vi "grab, fill rect, set:get pixel.vi"() -> ()   [LabVIEW 2011]
uses:
  <userlib>/labvvis/Rectangle.ctl
  <userlib>/labvvis/RGBA Pixel.ctl
  <userlib>/labvvis/New Image/New Image (RGBA).vi
  <userlib>/labvvis/Set Pixel/Set Pixel (RGBA).vi
  <userlib>/labvvis/Get Pixel/Get Pixel (RGBA).vi
  <userlib>/labvvis/labvvis.lvlib
panel:
  in  "Set Pixel":u8
  out "Error":string
  in  "Set Pixel":T1
  out "Get Pixel":u8
  out "Get Pixel":T1
  in  "Rectangle":T2
  in  "stop":bool
  out "Output":picture
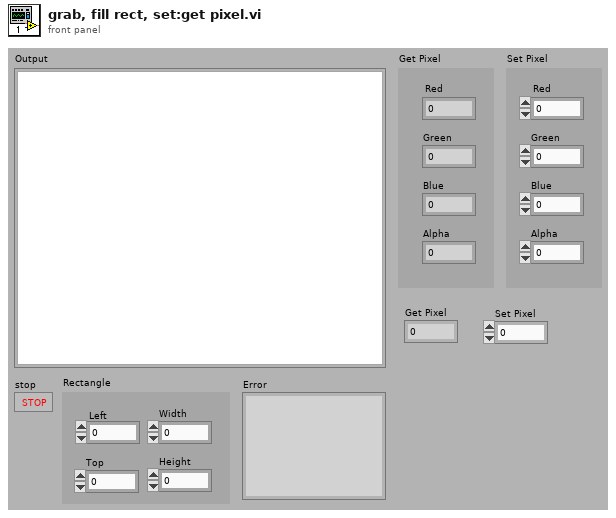
[diagram p1: front panel]
types:
  T1 = typedef "labvvis.lvlib/RGBA Pixel.ctl" = cluster{"Red ":u8, "Green":u8, "Blue":u8, "Alpha":u8}
  T2 = typedef "labvvis.lvlib/Rectangle.ctl" = cluster{"Left ":i32, "Top":i32, "Width":i32, "Height":i32}
  T3 = typedef "labvvis.lvlib/VVIS Image.ctl" = cluster{"Image ID":i16, "Channel ID":i16}
  T4 = typedef "imagedata.ctl" = cluster{"image type":i32, "image depth":i32, "image":u8[], "mask":u8[], "colors":u32[], "Rectangle":cluster{"left":i16, "top":i16, "right":i16, "bottom":i16}}
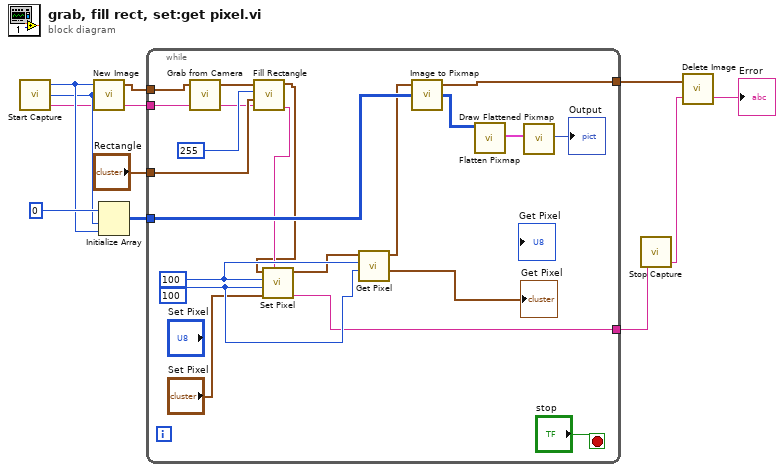
[diagram p0: block diagram]
diagram:
  n1 = call <userlib>:"Start Capture.vi"() -> ("Error"=w4:string, "Height"=w8:i32, "Width"=w9:i32)  [unwired: 3 in]
  n2 = call-poly <userlib>:"New Image.vi"("Error"=w4, "Height"=w8, "Width"=w9) -> ("Error"=w5:string, "VVIS Image"=w7:T3)  [unwired: 1 in]
  n3 = Initialize Array(0, w8, w9) -> (w11:i32[][])
  n4 = while {
    tunnel: w11 -> [w31]
    tunnel: [w29] -> w10
    tunnel: w7 -> [w27]
    tunnel: "Rectangle" -> [w24]
    tunnel: w5 -> [w17]
    tunnel: [w13] -> w3
    stop <- "stop" stop-if-true
    w22 = 100 ("Y")
    w23 = 100 ("X")
    n5 = call <userlib>:"Grab from Camera.vi"("Error"=w17, "Image"=w27) -> ("Error"=w19:string, "Image"=w26:T3)  [unwired: 1 in, 1 out]
    n6 = call <userlib>:"Fill Rectangle.vi"("Error"=w19, "Rectangle"=w24, "Value"=u8 255, "Image"=w26) -> ("Error"=w18:string, "Image"=w16:T3)  [unwired: 2 in]
    n7 = call-poly <userlib>:"Set Pixel.vi"("Error"=w18, "Pixel"="Set Pixel", "Y"=w22, "X"=w23, "Image"=w16) -> ("Error"=w13:string, "Image"=w15:T3)  [unwired: 2 in]
    n8 = call-poly <userlib>:"Get Pixel.vi"("Y"=w22, "X"=w23, "Image"=w15) -> ("Pixel"=→"Get Pixel":T1, "Image"=w14:T3)  [unwired: 2 in, 1 out]
    n9 = call <userlib>:"Image to Pixmap.vi"("Output Pixmap"=w31, "Image"=w14) -> ("Output Pixmap"=w30:u32[][], "Image"=w29:T3)  [unwired: 1 in, 1 out]
    n10 = call <vilib>:"Flatten Pixmap.vi"("24-bit pixmap"=w30) -> ("image data"=w33:T4)  [unwired: 10 in]
    n11 = call <vilib>:"Draw Flattened Pixmap.vi"("image data"=w33) -> ("new picture"=→"Output":picture)  [unwired: 8 in]
  }
  n12 = call <userlib>:"Stop Capture.vi"("Error"=w3) -> ("Error"=w2:string)  [unwired: 4 in]
  n13 = call <userlib>:"Delete Image.vi"("Error"=w2, "Image"=w10) -> ("Error"=→"Error":string)  [unwired: 1 in]
